vi "Get Exported 986x Support.vi"(8 "error in (no error)":errorcluster, 11 "Device Item Ref in":T2 format="%.0x") -> (0 "error out":errorcluster, 2 "986x Support":T1, 3 "Item Ref out":T2 format="%.0x")   [LabVIEW 2015, in "Diagnostics Addon System Explorer.lvlib"]
uses:
  Diagnostics Addon System Explorer.lvlib
  <vilib>/NI Veristand/Custom Device API/Custom Device Item Ref.ctl
  Types/Exported 986x Support.ctl
  <vilib>/NI Veristand/Custom Device API/Get Item Property (Path).vi
  <vilib>/NI Veristand/Custom Device API/Get Item Property (U16).vi
  <vilib>/NI Veristand/Custom Device API/Get Item Property (Boolean).vi
  Shared/SubVIs/GUID Lookup.vi
  <vilib>/NI Veristand/Custom Device API/Custom Device API.lvlib
  Shared/Diagnostics Addon Shared.lvlib
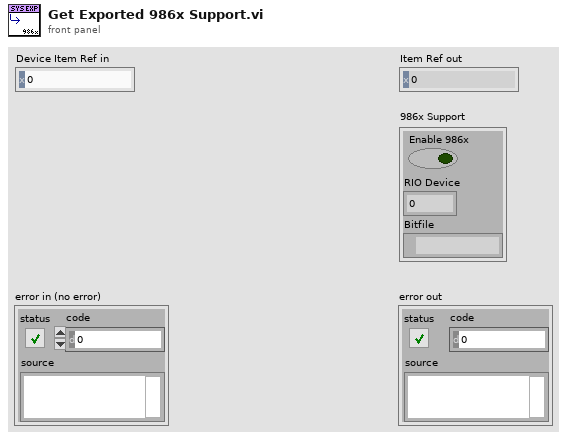
[diagram p1: front panel]
types:
  T1 = typedef "Diagnostics Addon System Explorer.lvlib/Exported 986x Support.ctl" = cluster{"Enable 986x":bool, "RIO Device":u16, "Bitfile":path}
  T2 = typedef "Custom Device API.lvlib/Custom Device Item Ref.ctl" = u64
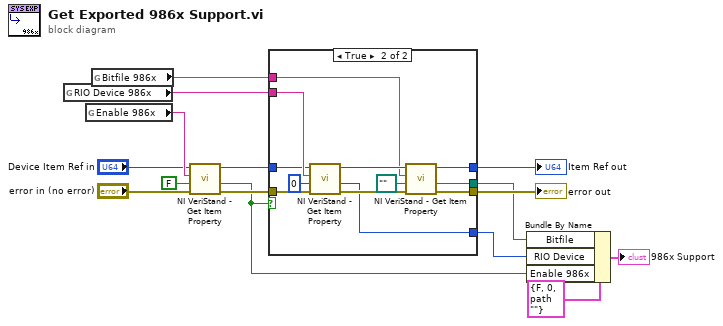
[diagram p0: block diagram]
diagram:
  n1 = global read "GUID Lookup.vi" "RIO Device 986x"() -> (w11:string)
  n2 = global read "GUID Lookup.vi" "Enable 986x"() -> (w9:string)
  n3 = global read "GUID Lookup.vi" "Bitfile 986x"() -> (w10:string)
  n4 = call-poly <vilib>:"NI VeriStand - Get Item Property.vi"("error in (no error)"="error in (no error)", "Default Value"=FALSE, "Property Name"=w9, "Item Ref in"="Device Item Ref in") -> ("error out"=w12:errorcluster, "Value"=w4:bool, "Item Ref out"=w13:T2)  [unwired: 4 in, 1 out]
  n5 = case shown="True" w4 {
    tunnel: w12 -> [w17 w29]
    tunnel: [w17 w25] -> w14
    tunnel: w11 -> [_ w28]
    tunnel: w10 -> [_ w22]
    tunnel: w13 -> [w16 w21]
    tunnel: [w16 w20] -> w15
    tunnel: [_ w19] -> w2
    tunnel: [_ w18] -> w3
    frame False {
    }
    frame True {
      n6 = call-poly <vilib>:"NI VeriStand - Get Item Property.vi"("error in (no error)"=w29, "Default Value"=u16 0, "Property Name"=w28, "Item Ref in"=w21) -> ("error out"=w26:errorcluster, "Value"=w19:u16, "Item Ref out"=w23:T2)  [unwired: 4 in, 1 out]
      n7 = call-poly <vilib>:"NI VeriStand - Get Item Property.vi"("error in (no error)"=w26, "Default Value"=path "", "Property Name"=w22, "Item Ref in"=w23) -> ("error out"=w25:errorcluster, "Value"=w18:path, "Item Ref out"=w20:T2)  [unwired: 4 in, 1 out]
    }
  }
  "Item Ref out" <- w15
  "error out" <- w14
  n8 = Bundle By Name(cluster=T1 {"Enable 986x"=FALSE, "RIO Device"=0, "Bitfile"=path ""}, "Bitfile"=w3, "RIO Device"=w2, "Enable 986x"=w4) -> (→"986x Support":T1)
